vi "公式写入.vi"(7 "公式":cluster{"X^2":dbl, "X":dbl, "b":dbl}, 8 "error in (no error)":errorcluster caption="错误输入（无错误）", 9 "量程":enum16{"低量程", "高量程"}(ring), 10 "测量模式":T1(ring), 11 "测量参数":enum16{"CODMn"}(ring)) -> (0 "error out":errorcluster caption="错误输出")   [LabVIEW 2016, in "斯坦道CODMn新电路板.lvlib"]
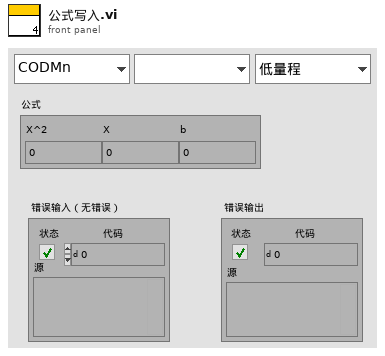
[diagram p1: front panel]
types:
  T1 = enum16{"", "水样测量", "标样核查", "零点核查", "跨度核查", "空白测试", "平行样测试", "加标回收"}
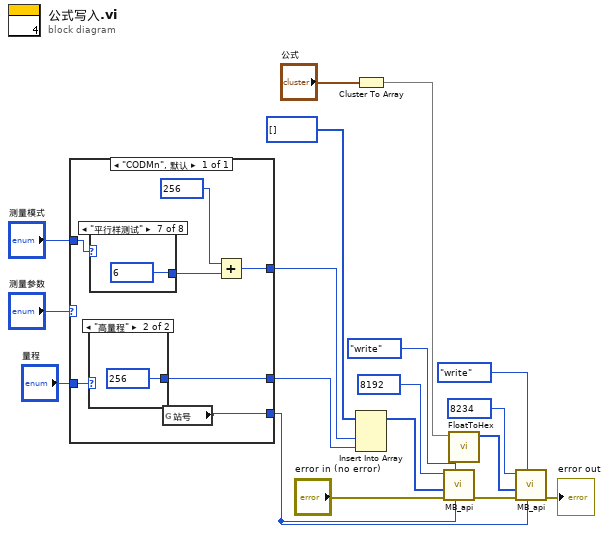
[diagram p0: block diagram]
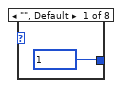
[diagram p2: hidden frame]
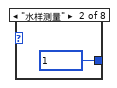
[diagram p3: hidden frame]
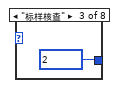
[diagram p4: hidden frame]
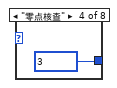
[diagram p5: hidden frame]
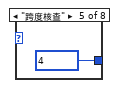
[diagram p6: hidden frame]
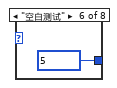
[diagram p7: hidden frame]
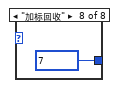
[diagram p8: hidden frame]
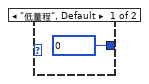
[diagram p9: hidden frame]
diagram:
  n1 = case shown="\"CODMn\", 默认" "测量参数" {
    tunnel: "测量模式" -> [w20]
    tunnel: "量程" -> [w25]
    tunnel: [w21] -> w6
    tunnel: [w22] -> w10
    tunnel: [w24] -> w9
    frame "CODMn", Default {
      n2 = case shown="\"高量程\"" w25 {
        tunnel: [u16 0 ("starting address") u16 256 ("starting address")] -> w24
        frame "低量程", Default {
        }
        frame "高量程" {
        }
      }
      n3 = case shown="\"平行样测试\"" w20 {
        tunnel: [u16 1 ("starting address") u16 1 ("starting address") u16 2 ("starting address") u16 3 ("starting address") u16 4 ("starting address") u16 5 ("starting address") u16 6 ("starting address") u16 7 ("starting address")] -> w19
        frame "", Default {
        }
        frame "水样测量" {
        }
        frame "标样核查" {
        }
        frame "零点核查" {
        }
        frame "跨度核查" {
        }
        frame "空白测试" {
        }
        frame "平行样测试" {
        }
        frame "加标回收" {
        }
      }
      n4 = global read "CODMn断电保存全局变量.vi" "站号"() -> (w21:u16)
      n5 = Add(x=u16 256 ("starting address"), y=w19) -> (x+y=w22:u16)
    }
  }
  n6 = Cluster To Array(cluster="公式") -> (array=w17:dbl[])
  n7 = Insert Into Array(array=u16[] [] ("数组"), new element #1=w10, new element #2=w9) -> (w2:u16[])  [unwired: 1 in]
  n8 = call "MB_api.vi"("Slave ID"=w6, "STEP"=enum16{"open", "read", "write", "close"}."write", "Error in"="error in (no error)", "values"=w2, "starting address"=u16 8192) -> ("error out"=w5:errorcluster)  [unwired: 4 in, 2 out]
  n9 = call "FloatToHex.vi"("浮点数"=w17) -> ("DCBA整形输出"=w1:u16[])  [unwired: 10 in]
  n10 = call "MB_api.vi"("Slave ID"=w6, "STEP"=enum16{"open", "read", "write", "close"}."write", "Error in"=w5, "values"=w1, "starting address"=u16 8234) -> ("error out"=→"error out":errorcluster)  [unwired: 4 in, 2 out]
